vi "Global 1.vi"() -> ()   [LabVIEW 2013]
panel:
  out "fail count":dbl
  out "dly value":dbl
  out "tmp dly lps":dbl
  out "COM port":refnum<visa-resource-name>="COM6"
  out "SAMPLES":dbl
  out "RATE(Hz)":dbl
  out "password":string
  out "C drive root path":path
  in  "Error In":errorcluster
  out "Mail Test":bool
  out "Mail Status":string
  out "MAIL SETTINGS":T1
  out "MAIL SELECT":T2
  in  "Network Drive":path
  out "LAB05-2 FILE":string
  out "LAB05-1 FILE":string
  out "LAB04-2 FILE":string
  out "LAB04-1 FILE":string
  out "LAB03-2 FILE":string
  out "LAB03-1 FILE":string
  out "LAB02-2 FILE":string
  out "LAB02-1 FILE":string
  out "LAB01-2 FILE":string
  out "LAB01-1 FILE":string
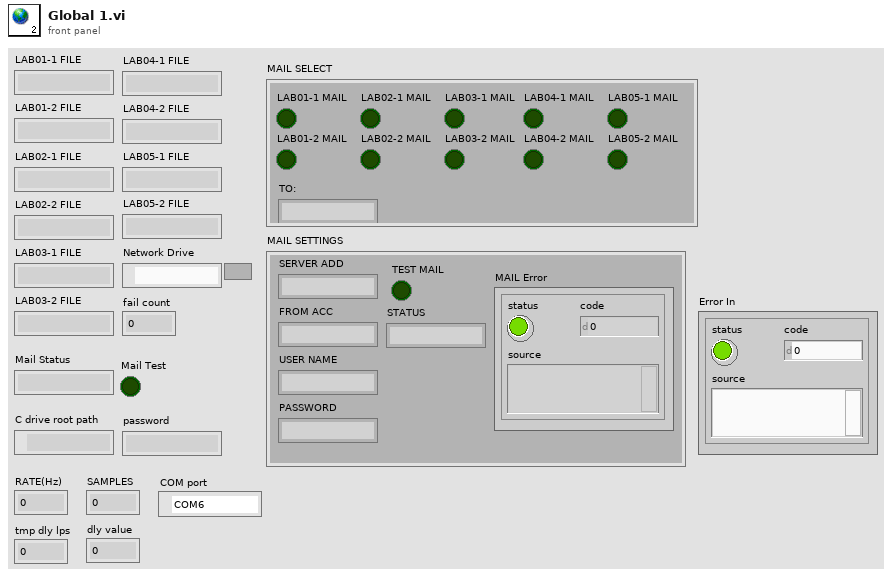
[diagram p1: front panel]
types:
  T1 = cluster{"SERVER ADD":string, "FROM ACC":string, "USER NAME":string, "PASSWORD":string, "TEST MAIL":bool, "STATUS":string, "MAIL Error":errorcluster}
  T2 = cluster{"LAB01-1 MAIL":bool, "LAB01-2 MAIL":bool, "LAB02-1 MAIL":bool, "LAB02-2 MAIL":bool, "LAB03-1 MAIL":bool, "LAB03-2 MAIL":bool, "LAB04-1 MAIL":bool, "LAB04-2 MAIL":bool, "LAB05-1 MAIL":bool, "LAB05-2 MAIL":bool, "TO:":string}
diagram:
